vi "Column Headers.vi"(8 "error in":errorcluster, 10 "column_header":string[](array[string]), 11 "stats in":refnum<class "stats.lvclass">) -> (0 "error out":errorcluster, 3 "stats out":refnum<class "stats.lvclass">)   [LabVIEW 2012, in "stats.lvclass"]
uses:
  stats.lvclass
  stats.lvclass/stats.ctl
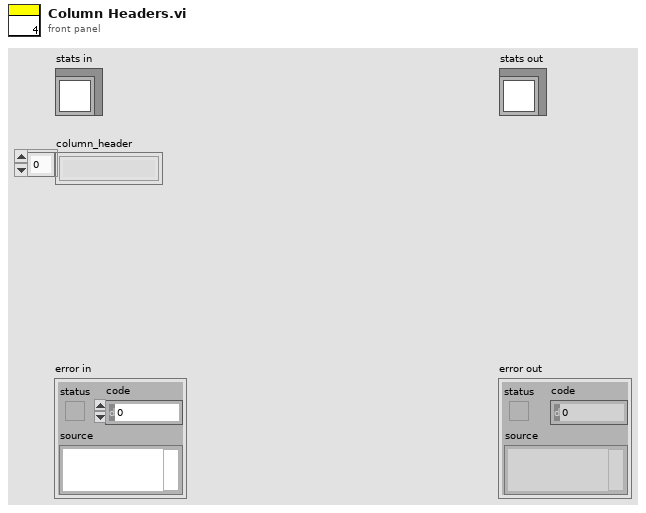
[diagram p1: front panel]
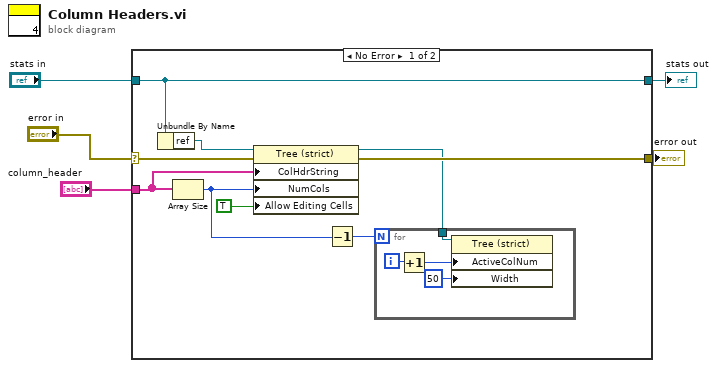
[diagram p0: block diagram]
diagram:
  n1 = case shown="No Error" "error in" {
    selector: "error in" -> [w12 w20]
    tunnel: [w11 w20] -> w4
    tunnel: [w14 w19] -> w2
    tunnel: "stats in" -> [w14 w19]
    tunnel: "column_header" -> [w10 _]
    frame No Error {
      n2 = Unbundle By Name(w14) -> ("ref"=w13:refnum<vi>)
      n3 = Array Size(array=w10) -> (size(s)=w8:i32)
      n4 = property class="Tree (strict)"(reference=w13, error in=w12, "ColHdrString"=w10, "NumCols"=w8, "Allow Editing Cells"=TRUE) -> (reference out=w6:refnum<vi>, error out=w11:errorcluster)
      n5 = Decrement(x=w8) -> (x-1=w7:i32)
      n6 = for {
        N: w7 -> [_]
        tunnel: w6 -> [w18]
        i -> [w17]
        n7 = Increment(x=w17) -> (x+1=w16:i32)
        n8 = property class="Tree (strict)"(reference=w18, "ActiveColNum"=w16, "Width"=50 ("Active Cell:Cell Size:Width")) -> ()  [unwired: 1 in, 2 out]
      }
    }
    frame Error {
    }
  }
  "error out" <- w4
  "stats out" <- w2
